vi "Xeryon Enter COM Port number.vi"() -> ()   [LabVIEW 2019]
panel:
  in  "OK":bool
  in  "COM-Port":string
  # "There was no valid preferences file found that holds a COM-port number.\n(..\\Preferences\\COM-port.txt)\n\nPlease enter a valid COM-port name. It will be saved in the correct location."
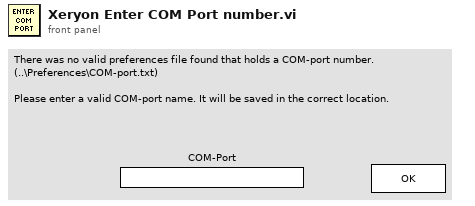
[diagram p1: front panel]
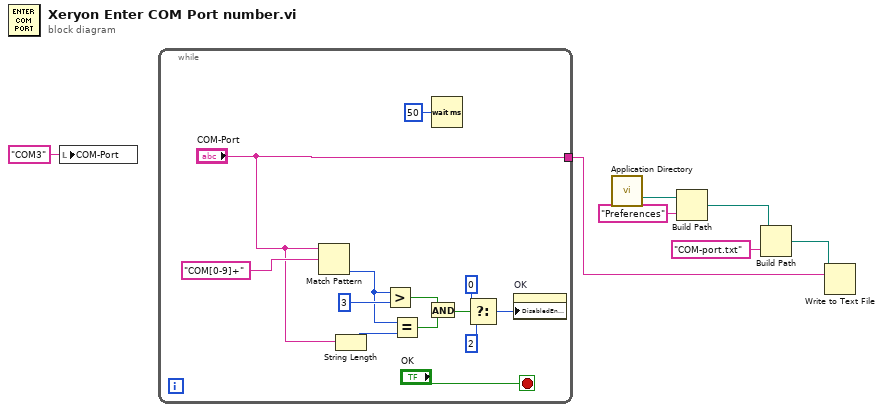
[diagram p0: block diagram]
diagram:
  n1 = local write "COM-Port"("COM3" ("COM-Port")) -> ()
  n2 = while {
    tunnel: ["COM-Port"] -> w1
    stop <- "OK" stop-if-true
    n3 = Match Pattern(string="COM-Port", regular expression="COM[0-9]+") -> (offset past match=w16:i32)  [unwired: 1 in, 3 out]
    n4 = String Length(string="COM-Port") -> (length=w15:i32)
    n5 = Greater?(x=w16, y=3) -> (0:w14:bool)
    n6 = Equal?(x=w16, y=w15) -> (x = y?=w13:bool)
    n7 = And(x=w14, y=w13) -> (x .and. y?=w12:bool)
    n8 = Wait (ms)(milliseconds to wait=u32 50) -> ()  [unwired: 1 out]
    n9 = Select(t=u32 0 ("milliseconds to wait"), s=w12, f=u32 2 ("milliseconds to wait")) -> (s? t:f=w11:u32)
    n10 = property on="OK" class="Bool"("DisabledEnum"=w11) -> ()  [unwired: 2 in, 2 out]
  }
  n11 = call <vilib>:"Application Directory.vi"() -> ("Application Directory"=w3:path)
  n12 = Build Path(base path=w3, name or relative path="Preferences") -> (appended path=w5:path)
  n13 = Build Path(base path=w5, name or relative path="COM-port.txt") -> (appended path=w2:path)
  n14 = Write to Text File(file (use dialog)=w2, text=w1) -> ()  [unwired: 2 in, 3 out]
